vi "AdvanceToNextProjectItem.vi"(8 "error in (no error)":errorcluster, 11 "BuildManager in":refnum<class "BuildManager.lvclass">) -> (0 "error out":errorcluster, 3 "BuildManager out":refnum<class "BuildManager.lvclass">)   [LabVIEW 2019, in "SolutionBuilder.lvlib" / "BuildManager.lvclass"]
uses:
  BuildManager.lvclass
  BuildManager.lvclass/BuildManager.ctl
  ProjectItem/ProjectItem.lvclass/ProjectItem.ctl
  ProjectItem/ProjectItem.lvclass
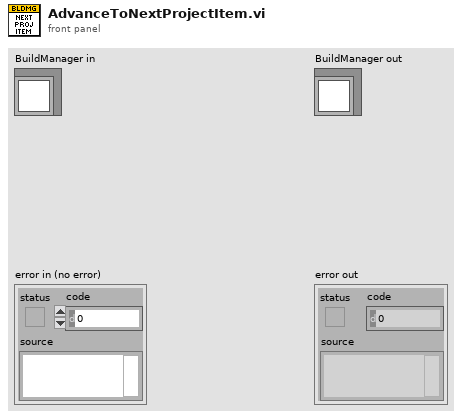
[diagram p1: front panel]
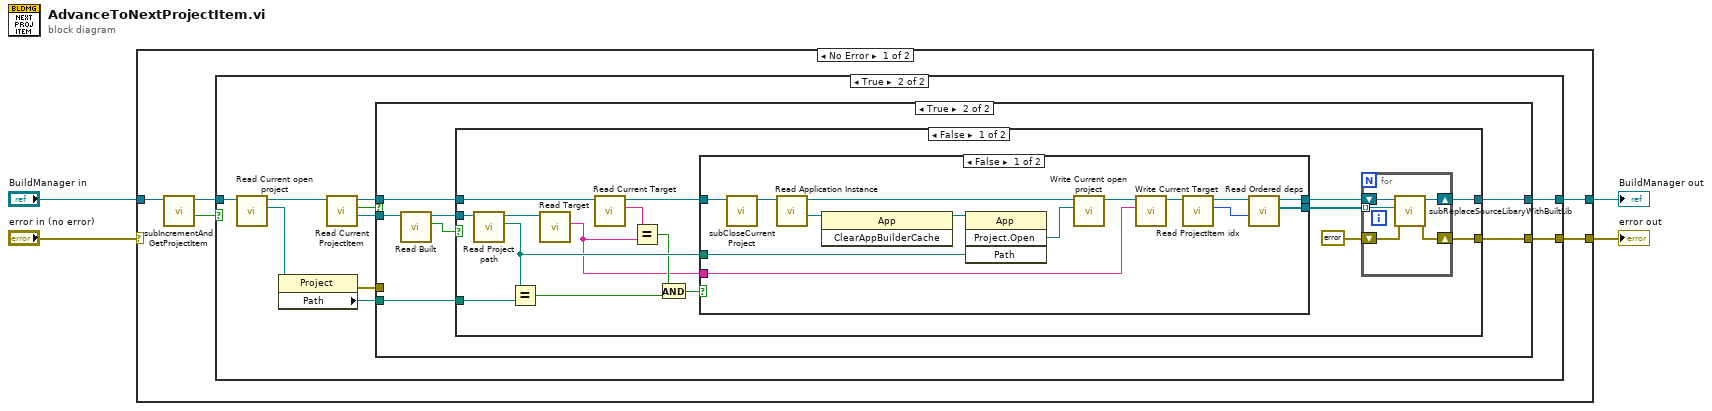
[diagram p0: block diagram]
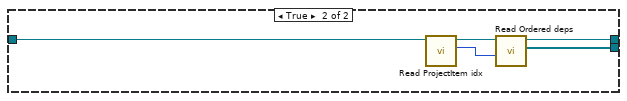
[diagram p4: hidden frame]
diagram:
  n1 = case shown="No Error" "error in (no error)" {
    selector: "error in (no error)" -> [_ w70]
    tunnel: [w9 w71] -> w4
    tunnel: "BuildManager in" -> [w8 w71]
    tunnel: [w5 w70] -> w1
    frame No Error {
      n2 = call "subIncrementAndGetProjectItem.vi"("BuildManager in"=w8) -> ("Valid"=w6:bool, "BuildManager out"=w7:refnum<class "BuildManager.lvclass">)  [unwired: 8 in, 1 out]
      n3 = case shown="True" w6 {
        tunnel: [w10 w19] -> w9
        tunnel: w7 -> [w10 w17]
        tunnel: [_ w12] -> w5
        frame False {
        }
        frame True {
          n4 = call-dynamic "Read Current open project.vi"("BuildManager in"=w17) -> ("Current open project"=w18:refnum<vi>, "BuildManager out"=w16:refnum<class "BuildManager.lvclass">)  [unwired: 9 in]
          n5 = property class="Project"(reference=w18) -> (error out=w11:errorcluster, "Path"=w20:path)  [unwired: 1 in, 1 out]
          n6 = call-dynamic "Read Current ProjectItem.vi"("BuildManager in"=w16) -> ("Current ProjectItem"=w13:refnum<class "ProjectItem.lvclass">, "Valid"=w14:bool, "BuildManager out"=w15:refnum<class "BuildManager.lvclass">)  [unwired: 7 in, 1 out]
          n7 = case shown="True" w14 {
            tunnel: w20 -> [_ w28]
            tunnel: [w21 w27] -> w19
            tunnel: w15 -> [w21 w26]
            tunnel: w13 -> [_ w24]
            tunnel: [_ w23] -> w12
            tunnel: w11 -> [_ _]
            frame False {
            }
            frame True {
              n8 = call-dynamic "Read Built.vi"("ProjectItem in"=w24) -> ("Built"=w22:bool, "ProjectItem out"=w25:refnum<class "ProjectItem.lvclass">)  [unwired: 9 in]
              n9 = case shown="False" w22 {
                tunnel: w28 -> [w44 _]
                tunnel: [w29 w69] -> w27
                tunnel: w26 -> [w37 w69]
                tunnel: w25 -> [w41 _]
                tunnel: [w39 _] -> w23
                frame False {
                  n10 = call-dynamic "Read Project path.vi"("ProjectItem in"=w41) -> ("Project path"=w43:path, "ProjectItem out"=w38:refnum<class "ProjectItem.lvclass">)  [unwired: 9 in]
                  n11 = Equal?(x=w43, y=w44) -> (x = y?=w33:bool)
                  n12 = call "Read Target.vi"("ProjectItem in"=w38) -> ("Target"=w31:string)  [unwired: 9 in, 1 out]
                  n13 = call "Read Current Target.vi"("BuildManager in"=w37) -> ("Current Target"=w35:string, "BuildManager out"=w36:refnum<class "BuildManager.lvclass">)  [unwired: 9 in]
                  n14 = Equal?(x=w35, y=w31) -> (x = y?=w34:bool)
                  n15 = And(x=w34, y=w33) -> (x .and. y?=w32:bool)
                  n16 = case shown="False" w32 {
                    tunnel: w36 -> [w58 w63]
                    tunnel: [w55 w61] -> w30
                    tunnel: w43 -> [w57 _]
                    tunnel: [w53 w60] -> w42
                    tunnel: w31 -> [w50 _]
                    frame False {
                      n17 = call "subCloseCurrentProject.vi"("BuildManager in"=w58) -> ("BuildManager out"=w49:refnum<class "BuildManager.lvclass">)  [unwired: 9 in, 1 out]
                      n18 = call-dynamic "Read Application Instance.vi"("BuildManager in"=w49) -> ("Application Instance"=w46:refnum<vi>, "BuildManager out"=w48:refnum<class "BuildManager.lvclass">)  [unwired: 9 in]
                      n19 = invoke class="App" method="ClearAppBuilderCache"(reference=w46) -> (reference out=w45:refnum<vi>)  [unwired: 2 in, 2 out]
                      n20 = invoke class="App" method="Project.Open"(reference=w45, "Path"=w57) -> ("Project:Open"=w47:refnum<vi>)  [unwired: 2 in, 3 out]
                      n21 = call-dynamic "Write Current open project.vi"("Current open project"=w47, "BuildManager in"=w48) -> ("BuildManager out"=w52:refnum<class "BuildManager.lvclass">)  [unwired: 9 in]
                      n22 = call "Write Current Target.vi"("Current Target"=w50, "BuildManager in"=w52) -> ("BuildManager out"=w51:refnum<class "BuildManager.lvclass">)  [unwired: 9 in]
                      n23 = call-dynamic "Read ProjectItem idx.vi"("BuildManager in"=w51) -> ("ProjectItem idx"=w54:i32, "BuildManager out"=w56:refnum<class "BuildManager.lvclass">)  [unwired: 9 in]
                      n24 = call-dynamic "Read Ordered deps.vi"("length (-1)"=w54, "BuildManager in"=w56) -> ("Ordered deps"=w53:refnum<class "ProjectItem.lvclass">[], "BuildManager out"=w55:refnum<class "BuildManager.lvclass">)  [unwired: 8 in]
                    }
                    frame True {
                      n25 = call-dynamic "Read ProjectItem idx.vi"("BuildManager in"=w63) -> ("ProjectItem idx"=w59:i32, "BuildManager out"=w62:refnum<class "BuildManager.lvclass">)  [unwired: 9 in]
                      n26 = call-dynamic "Read Ordered deps.vi"("length (-1)"=w59, "BuildManager in"=w62) -> ("Ordered deps"=w60:refnum<class "ProjectItem.lvclass">[], "BuildManager out"=w61:refnum<class "BuildManager.lvclass">)  [unwired: 8 in]
                    }
                  }
                  n27 = for {
                    shift-right: [w66] -> w29
                    shift-left: w30 -> [w67]
                    tunnel: w42 -> [w68] mode=indexing
                    shift-right: [w65] -> w39
                    shift-left: errorcluster {"status"=FALSE, "code"=0, "source"=""} ("error out") -> [w64]
                    n28 = call "subReplaceSourceLibaryWithBuiltLib.vi"("error in (no error)"=w64, "ProjectItem in"=w68, "BuildManager in"=w67) -> ("error out"=w65:errorcluster, "BuildManager out"=w66:refnum<class "BuildManager.lvclass">)  [unwired: 7 in]
                  }
                }
                frame True {
                }
              }
            }
          }
        }
      }
    }
    frame Error {
    }
  }
  "error out" <- w1
  "BuildManager out" <- w4
